vi "CThread Autonomous Template.vi"() -> ()   [LabVIEW 2010]
uses:
  CLIB/CThread/XNodes/initializernode/CThread Initializer.xnode
  <vilib>/NXT/Remote Library/File Access/NXT_FileType.ctl
  CLIB/CThread/Core/CThread Governor.vi
  Process All FTC Functions.vi
  <vilib>/NXT/Dual Mode Library/Waits/Wait_Num(msec).vi
  Remote Interface/internal/Polymorphic Selections/NXTLeft.vi
  <vilib>/NXT/Dual Mode Library/Display/drawText.vi
  <vilib>/NXT/Dual Mode Library/Display/clearDisplay.vi
  FTC.lvlib
  Components/Components.lvlib
  Remote Interface/Remote Interface.lvlib
  CLIB/CThread/CThread.lvlib
panel:
  out "Autonomous ID":i32
  out "Enabled":bool
  out "Enabled?":enum16{"Disabled", "Enabled"}(ring)
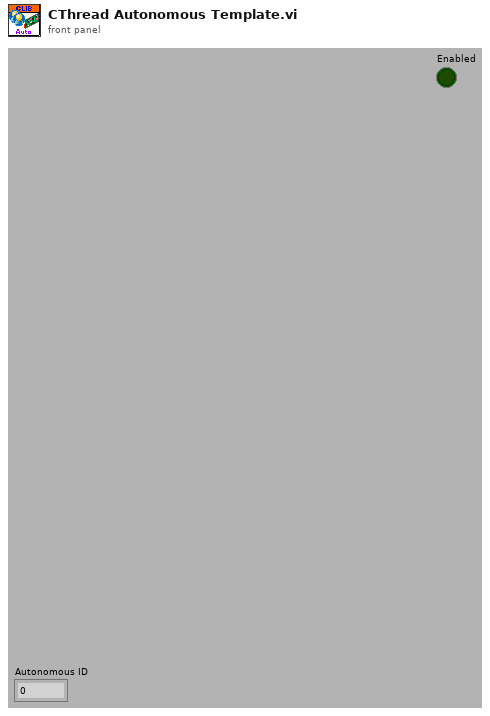
[diagram p1: front panel]
types:
  T1 = typedef "LVHSConnector.ctl" = cluster{"Hardware":string, "Flattened String":string}
  T2 = cluster{"ID":u32, "Display Character":string, "Option Message":string}[]
  T3 = typedef "NXT_FileType.ctl" = u16
  T4 = typedef "SequenceBoolean.ctl" = bool
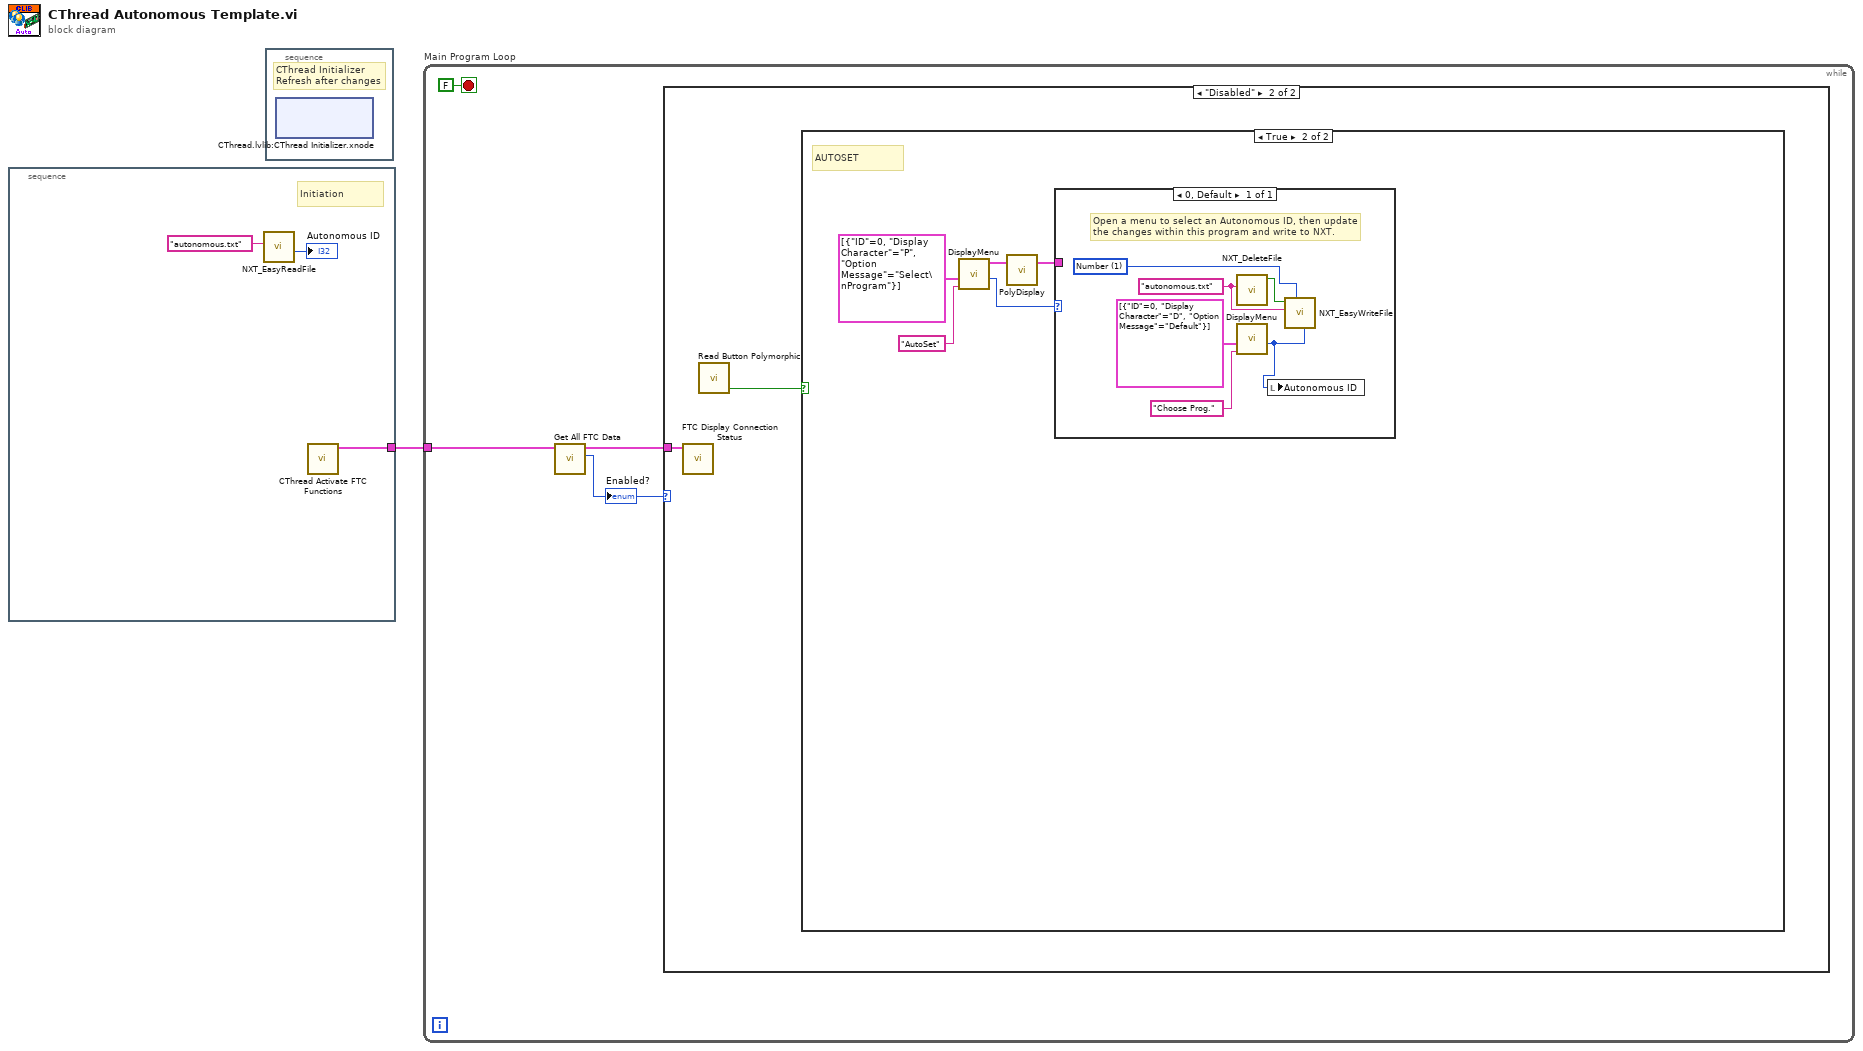
[diagram p0: block diagram]
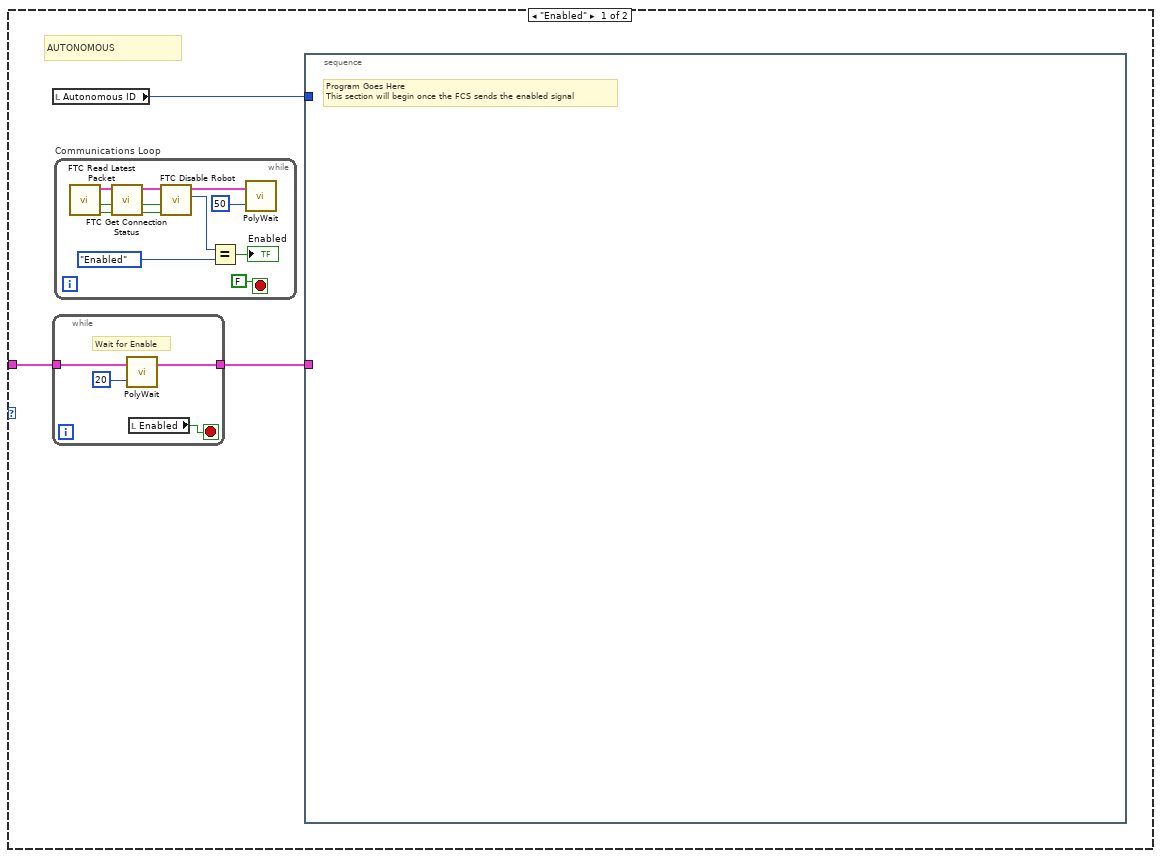
[diagram p2: hidden frame]
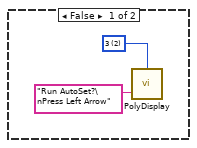
[diagram p3: hidden frame]
diagram:
  n1 = stacked-sequence {
    tunnel: [w2] -> w1
    frame #0 {
      # "Initiation"
      n2 = call <vilib>:"NXT_EasyReadFile.vi"("Filename"="autonomous.txt") -> ("Number"=→"Autonomous ID":i32)  [unwired: 7 in, 3 out]
      n3 = call "CThread Activate FTC Functions.vi"() -> ("NXT"=w2:T1)  [unwired: 11 in]
    }
  }
  n4 = stacked-sequence {
    frame #0 {
      # "CThread Initializer\nRefresh after changes"
      n5 = xnode "CThread.lvlib:CThread Initializer.xnode"() -> ()
    }
  }
  n6 = while "Main Program Loop" {
    tunnel: w1 -> [w20]
    stop <- FALSE stop-if-true
    n7 = call "Get All FTC Data.vi"("NXT"=w20) -> ("Enabled?"=w18:enum16{"Disabled", "Enabled"}, "NXT"=w19:T1)  [unwired: 3 in, 6 out]
    "Enabled?" <- w18
    n8 = case "disableCase" shown="\"Disabled\"" w18 {
      tunnel: w19 -> [w24 w42]
      frame "Enabled" {
        # "AUTONOMOUS"
        n9 = local read "Autonomous ID"() -> (w22:i32)
        n10 = while {
          tunnel: [w27] -> w23
          tunnel: w24 -> [w26]
          stop <- w25 stop-if-true
          # "Wait for Enable"
          n11 = call-poly <vilib>:"PolyWait.vi"("Time (100 msec)"=u32 20 ("Time (msec)"), "NXT"=w26) -> ("NXT"=w27:T1)  [unwired: 2 in]
          n12 = local read "Enabled"() -> (w25:bool)
        }
        n13 = while "Communications Loop" {
          stop <- FALSE stop-if-true
          n14 = call <vilib>:"FTC Read Latest Packet.vi"() -> ("Packet Received?"=w38:bool, "Stopped?"=w37:bool, "NXT"=w40:T1)  [unwired: 6 in, 3 out]
          n15 = call <vilib>:"FTC Get Connection Status.vi"("Packet Received?"=w38, "Stopped?"=w37, "NXT"=w40) -> ("Online?"=w30:bool, "Stopped?"=w31:bool, "NXT"=w39:T1)  [unwired: 5 in]
          n16 = call <vilib>:"FTC Disable Robot.vi"("Online?"=w30, "Stopped?"=w31, "NXT"=w39) -> ("Enabled?"=w29:enum16{"Disabled", "Enabled"}, "NXT"=w35:T1)  [unwired: 3 in]
          n17 = Equal?(x=w29, y=enum16{"Disabled", "Enabled"}."Enabled") -> (x = y?=→"Enabled":bool)
          n18 = call-poly <vilib>:"PolyWait.vi"("Time (100 msec)"=u32 50 ("Time (msec)"), "NXT"=w35) -> ()  [unwired: 2 in, 1 out]
        }
        n19 = stacked-sequence {
          tunnel: w23 -> [_]
          tunnel: w22 -> [_]
          frame #0 {
            # "Program Goes Here\nThis section will begin once the FCS sends the enabled signal"
          }
        }
      }
      frame "Disabled" {
        n20 = call <vilib>:"FTC Display Connection Status.vi"("NXT"=w42) -> ()  [unwired: 10 in, 1 out]
        n21 = call-poly "Read Button Polymorphic.vi"() -> ("Pressed?"=w41:bool)  [unwired: 7 in]
        n22 = case shown="True" w41 {
          frame False {
            w43 = i16 2 items=["1", "2", "3", "4", "5", "6", "7", "8"] ("Line")
            n23 = call-poly <vilib>:"PolyDisplay.vi"("Text"="Run AutoSet?\nPress Left Arrow", "Line"=w43) -> ()  [unwired: 2 in, 1 out]
          }
          frame True {
            # "AUTOSET"
            n24 = call "DisplayMenu.vi"("Menu Message"="AutoSet", "Options"=T2 [{"ID"=0, "Display Character"="P", "Option Message"="Select\nProgram"}]) -> ("Selected ID"=w49:u32, "NXT"=w48:T1)  [unwired: 6 in]
            n25 = call-poly <vilib>:"PolyDisplay.vi"("NXT"=w48) -> ("NXT"=w47:T1)  [unwired: 3 in]
            n26 = case shown="0, Default" w49 {
              tunnel: w47 -> [_]
              frame 0, Default {
                w53 = "autonomous.txt"
                w55 = T3 1 items=["Text", "Number"] ("Type")
                # "Open a menu to select an Autonomous ID, then update\nthe changes within this program and write to NXT."
                n27 = call <vilib>:"NXT_DeleteFile.vi"("Filename"=w53) -> ("Sequence Flow out"=w54:T4)  [unwired: 9 in, 1 out]
                n28 = call "DisplayMenu.vi"("Menu Message"="Choose Prog.", "Options"=T2 [{"ID"=0, "Display Character"="D", "Option Message"="Default"}]) -> ("Selected ID"=w50:u32)  [unwired: 6 in, 1 out]
                n29 = local write "Autonomous ID"(w50) -> ()
                n30 = call <vilib>:"NXT_EasyWriteFile.vi"("Number"=w50, "Type"=w55, "Filename"=w53, "Sequence Flow in"=w54) -> ()  [unwired: 6 in, 2 out]
              }
            }
          }
        }
      }
    }
  }
